vi "2-Opt(Zobolas) Neighborhood.vi"(11 "Schedule in":u16[](array[numeric])) -> (3 "Schedule out":u16[](array[numeric]))   [LabVIEW 2013]
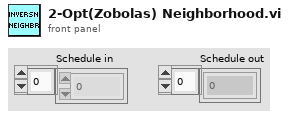
[diagram p1: front panel]
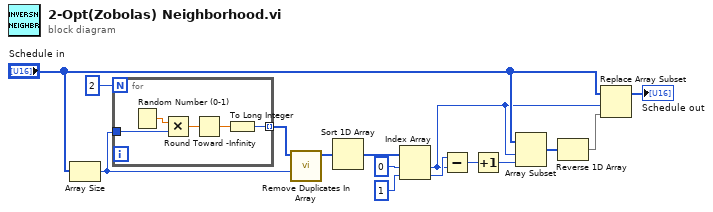
[diagram p0: block diagram]
diagram:
  n1 = Array Size(array="Schedule in") -> (size(s)=w11:i32)
  n2 = for {
    N: 2 -> [_]
    tunnel: w11 -> [w17]
    tunnel: [w16] -> w12 mode=indexing
    n3 = Random Number (0-1)() -> (number: 0 to 1=w20:dbl)
    n4 = Multiply(x=w20, y=w17) -> (x*y=w19:dbl)
    n5 = Round Toward -Infinity(1:w19) -> (0:w18:dbl)
    n6 = To Long Integer(number=w18) -> (32bit integer=w16:i32)
  }
  n7 = call "Remove Duplicates In Array.vi"("Max Index Bound"=w11, "Random Numbers Array"=w12) -> ("Random Numbers Array without Duplicates"=w8:i32[])  [unwired: 9 in]
  n8 = Sort 1D Array(array=w8) -> (sorted array=w7:i32[])
  n9 = Index Array(array=w7, index #1=0 ("index"), index #2=1 ("index")) -> (element #1=w5:i32, element #2=w6:i32)
  n10 = Subtract(x=w6, y=w5) -> (x-y=w2:i32)
  n11 = Increment(x=w2) -> (x+1=w1:i32)
  n12 = Array Subset(array="Schedule in", index=w5, length=w1) -> (w4:u16[])
  n13 = Reverse 1D Array(array=w4) -> (reversed array=w3:u16[])
  n14 = Replace Array Subset(array="Schedule in", new element=w3, index=w5) -> (→"Schedule out":u16[])
